vi "DotProduct.vi"(1 "Vec2 b in":refnum<class "Vector2.lvclass">, 2 "Vec2 a in":refnum<class "Vector2.lvclass">) -> (0 "Product out":dbl)   [LabVIEW 2022 SP3, in "Vector2.lvclass"]
uses:
  Vector2.lvclass
  Vector2.lvclass/Vector2.ctl
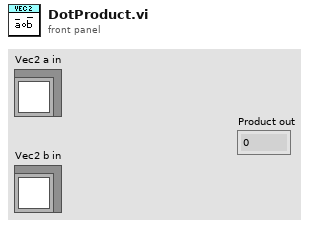
[diagram p1: front panel]
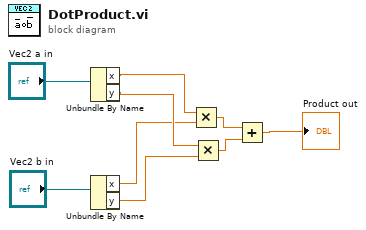
[diagram p0: block diagram]
diagram:
  n1 = Unbundle By Name("Vec2 a in") -> ("x"=w7:dbl, "y"=w6:dbl)
  n2 = Unbundle By Name("Vec2 b in") -> ("x"=w5:dbl, "y"=w4:dbl)
  n3 = Multiply(x=w7, y=w5) -> (x*y=w3:dbl)
  n4 = Multiply(x=w6, y=w4) -> (x*y=w2:dbl)
  n5 = Add(x=w3, y=w2) -> (x+y=→"Product out":dbl)
